vi "Unflatten.vi"(8 "error in (no error)":errorcluster, 11 "anritsu reader in":refnum<class "anritsu reader.lvclass">) -> (0 "error out":errorcluster, 3 "anritsu reader out":refnum<class "anritsu reader.lvclass">)   [LabVIEW 2009, in "anritsu reader.lvclass"]
uses:
  anritsu reader.lvclass
  Reader/Reader.lvclass
  Global/File Locations.vi
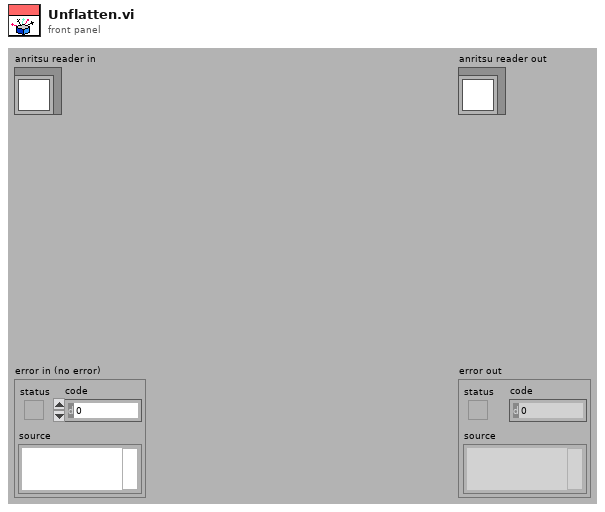
[diagram p1: front panel]
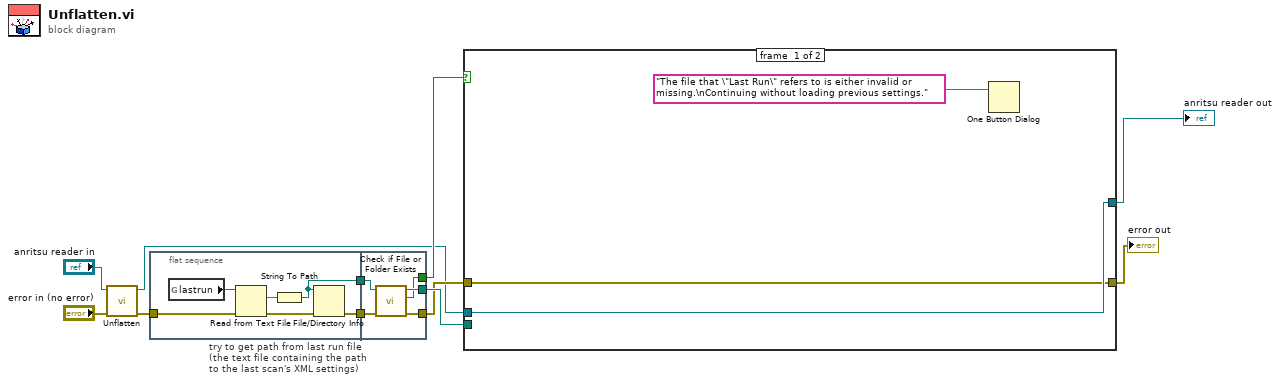
[diagram p0: block diagram]
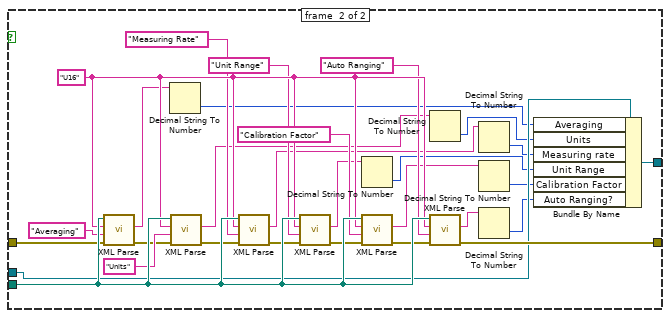
[diagram p2: hidden frame]
diagram:
  n1 = call-parent "Unflatten.vi"("error in (no error)"="error in (no error)", "Reader in"="anritsu reader in") -> ("error out"=w7:errorcluster, "Reader out"=w3:refnum<class "anritsu reader.lvclass">)  [unwired: 8 in]
  n2 = flat-sequence "try to get path from last run file\n(the text file containing the path\nto the last scan's XML settings)" {
    tunnel: w7 -> [w12]
    tunnel: [w17] -> w9
    tunnel: [w13] -> w8
    tunnel: [w21] -> w4
    tunnel: [w22] -> w5
    tunnel: w9 -> [w19]
    tunnel: w8 -> [w20]
    tunnel: [w18] -> w6
    frame #0 {
      n3 = global read "File Locations.vi" "lastrun"() -> (w15:path)
      n4 = Read from Text File(file (use dialog)=w15, error in=w12) -> (text=w16:string, error out=w14:errorcluster)  [unwired: 4 out]
      n5 = String To Path(string=w16) -> (path=w17:path)
      n6 = File/Directory Info(path=w17, error in=w14) -> (error out=w13:errorcluster)  [unwired: 6 out]
    }
    frame #1 {
      n7 = call <vilib>:"Check if File or Folder Exists.vi"("error in (no error)"=w20, "path"=w19) -> ("error out"=w21:errorcluster, "file or folder exists?"=w18:bool, "dup path"=w22:path)  [unwired: 7 in]
    }
  }
  n8 = case shown="True" w6 {
    tunnel: w3 -> [w24 w39]
    tunnel: [w24 w38] -> w2
    tunnel: w5 -> [_ w54]
    tunnel: w4 -> [w23 w46]
    tunnel: [w23 w40] -> w1
    frame #0 {
      n9 = One Button Dialog(message="The file that \"Last Run\" refers to is either invalid or missing.\nContinuing without loading previous settings.") -> ()  [unwired: 1 in, 1 out]
    }
    frame #1 {
      w53 = "U16"
      n10 = call "XML Parse.vi"("error in (no error)"=w46, "Name String"="Averaging", "Type String"=w53, "Path"=w54) -> ("error out"=w45:errorcluster, "String Out"=w37:string)  [unwired: 6 in]
      n11 = Decimal String To Number(string=w37) -> (number=w36:i32)  [unwired: 2 in, 1 out]
      n12 = call "XML Parse.vi"("error in (no error)"=w45, "Name String"="Units", "Type String"=w53, "Path"=w54) -> ("error out"=w44:errorcluster, "String Out"=w35:string)  [unwired: 6 in]
      n13 = call "XML Parse.vi"("error in (no error)"=w44, "Name String"="Measuring Rate", "Type String"=w53, "Path"=w54) -> ("error out"=w43:errorcluster, "String Out"=w33:string)  [unwired: 6 in]
      n14 = call "XML Parse.vi"("error in (no error)"=w43, "Name String"="Unit Range", "Type String"=w53, "Path"=w54) -> ("error out"=w42:errorcluster, "String Out"=w31:string)  [unwired: 6 in]
      n15 = Decimal String To Number(string=w31) -> (number=w30:i32)  [unwired: 2 in, 1 out]
      n16 = call "XML Parse.vi"("error in (no error)"=w42, "Name String"="Calibration Factor", "Type String"=w53, "Path"=w54) -> ("error out"=w41:errorcluster, "String Out"=w29:string)  [unwired: 6 in]
      n17 = Decimal String To Number(string=w35) -> (number=w34:i32)  [unwired: 2 in, 1 out]
      n18 = call "XML Parse.vi"("error in (no error)"=w41, "Name String"="Auto Ranging", "Type String"=w53, "Path"=w54) -> ("error out"=w40:errorcluster, "String Out"=w27:string)  [unwired: 6 in]
      n19 = Decimal String To Number(string=w33) -> (number=w32:i32)  [unwired: 2 in, 1 out]
      n20 = Decimal String To Number(string=w29) -> (number=w28:i32)  [unwired: 2 in, 1 out]
      n21 = Decimal String To Number(string=w27) -> (number=w26:i32)  [unwired: 2 in, 1 out]
      n22 = Bundle By Name(cluster=w39, "Averaging"=w36, "Units"=w34, "Measuring rate"=w32, "Unit Range"=w30, "Calibration Factor"=w28, "Auto Ranging?"=w26) -> (w38:refnum<class "anritsu reader.lvclass">)
    }
  }
  "error out" <- w1
  "anritsu reader out" <- w2
